vi "TableGluing.vi"() -> ()   [LabVIEW 2015]
uses:
  GlobalPath.vi
  GlobalData.vi
  GlobalVi.vi
panel:
  in  "Done with gluing?":bool
  in  "ptfe 7":bool caption="Remove the parchment covers from on top of the PCBs"
  in  "ptfe 6":bool caption="Remove the frames, cooling bars and honeycombs from on top of \nthe PCBs on the table"
  in  "Done?":bool
  in  "ptfe 5":bool caption="Open the vi with the gluing instructions"
  in  "ptfe 4":bool caption="Position the cartridge on the glue machine housing"
  in  "ptfe 3":bool caption="Mount the dispenser on the glue cartridge"
  in  "ptfe 2":bool caption="Position parchment covers to protect the reference plates and external \nparts of the 5 PCBs"
  # "Gluing on Table"
  # "Start gluing process"
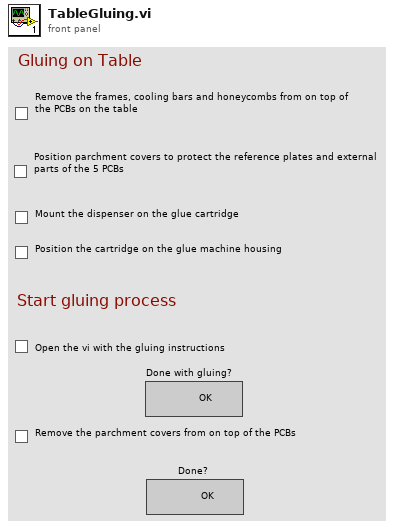
[diagram p1: front panel]
types:
  T1 = enum16{"open", "replace", "create", "open or create", "replace or create", "replace or create with confirmation"}
  T2 = enum32{"Bad", "Idle", "Run top level", "Running"}
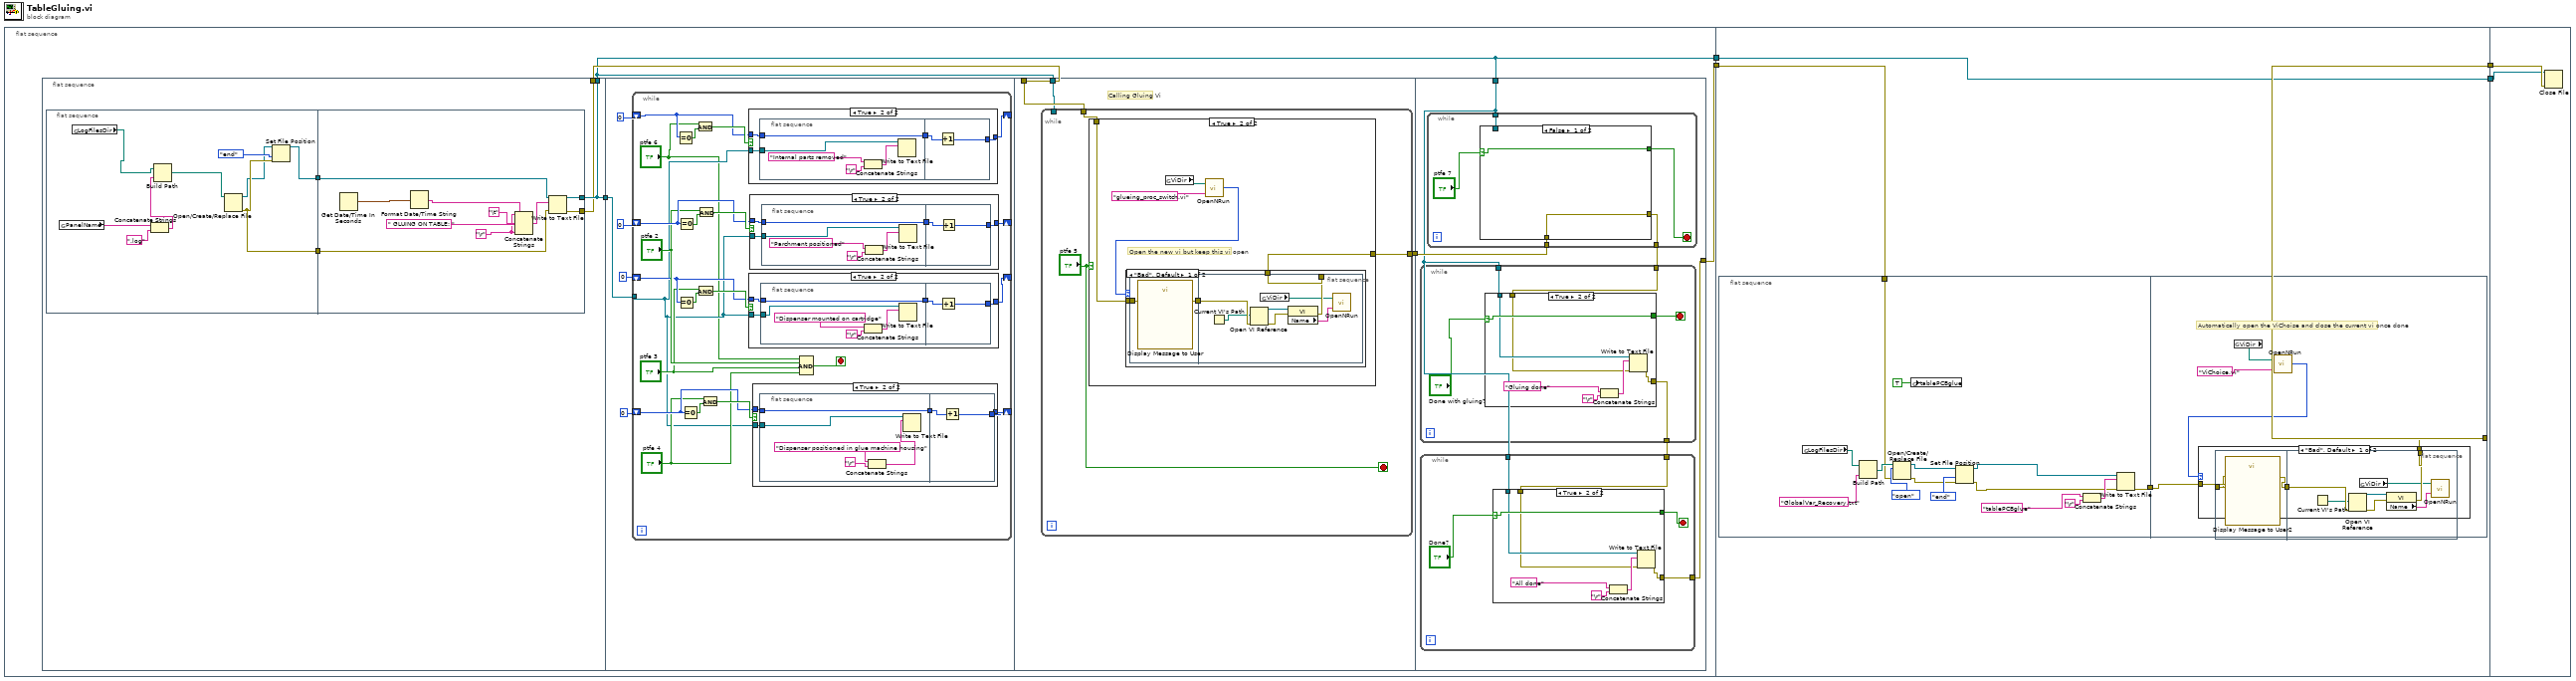
[diagram p0: block diagram]
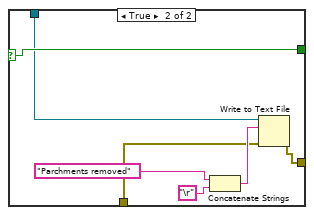
[diagram p9: hidden frame]
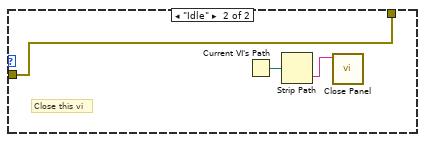
[diagram p11: hidden frame]
diagram:
  n1 = flat-sequence {
    tunnel: [w6] -> w3
    tunnel: [w5] -> w1
    tunnel: [w183] -> w4
    tunnel: w3 -> [w182]
    tunnel: [w182] -> w2
    tunnel: w1 -> [w180]
    tunnel: w4 -> [w220]
    tunnel: w2 -> [w219]
    frame #0 {
      n2 = flat-sequence {
        tunnel: [w12] -> w9
        tunnel: [w12] -> w6
        tunnel: [w11] -> w8
        tunnel: w9 -> [w37]
        tunnel: w8 -> [w110]
        tunnel: w6 -> [w108]
        tunnel: [w109] -> w7
        tunnel: [w134] -> w5
        tunnel: w7 -> [w137]
        tunnel: w6 -> [w133]
        frame #0 {
          n3 = flat-sequence {
            tunnel: [w15] -> w13
            tunnel: [w17] -> w10
            tunnel: w13 -> [w28]
            tunnel: [w27] -> w12
            tunnel: [w26] -> w11
            tunnel: w10 -> [w25]
            frame #0 {
              n4 = global read "GlobalData.vi" "PanelName"() -> (w21:string)
              n5 = global read "GlobalPath.vi" "LogFilesDir"() -> (w14:path)
              n6 = Concatenate Strings(w21, ".log") -> (w20:string)
              n7 = Build Path(base path=w14, name or relative path=w20) -> (appended path=w19:path)
              n8 = Open/Create/Replace File(file path (use dialog)=w19) -> (refnum out=w16:refnum<file>, error out=w17:errorcluster)  [unwired: 5 in, 1 out]
              n9 = Set File Position(refnum=w16, from (0:start)=enum16{"start", "end", "current"}."end", error in=w17) -> (refnum out=w15:refnum<file>)  [unwired: 1 in, 1 out]
            }
            frame #1 {
              w23 = "\r"
              n10 = Get Date/Time In Seconds() -> (seconds since 1Jan1904=w24:timestamp)
              n11 = Format Date/Time String(seconds (now)=w24) -> (date/time string=w30:string)  [unwired: 2 in]
              n12 = Concatenate Strings(w23, w30, "\t", " GLUING ON TABLE: ", w23) -> (w29:string)
              n13 = Write to Text File(file (use dialog)=w28, text=w29, error in=w25) -> (refnum out=w27:refnum<file>, error out=w26:errorcluster)  [unwired: 1 in, 1 out]
            }
          }
        }
        frame #1 {
          n14 = while {
            tunnel: w37 -> [w39]
            shift-right: [w55] -> _
            shift-left: 0 -> [w56]
            shift-right: [w46] -> _
            shift-left: 0 -> [w51]
            shift-right: [w45] -> _
            shift-left: 0 -> [w47]
            shift-right: [w41] -> _
            shift-left: 0 -> [w40]
            stop <- w59 stop-if-true
            n15 = Equal To 0?(x=w40) -> (x = 0?=w43:bool)
            n16 = Equal To 0?(x=w51) -> (x = 0?=w53:bool)
            n17 = Equal To 0?(x=w56) -> (x = 0?=w58:bool)
            n18 = Equal To 0?(x=w47) -> (x = 0?=w49:bool)
            n19 = And(x="ptfe 6", y=w43) -> (x .and. y?=w42:bool)
            n20 = And(x="ptfe 3", y=w53) -> (x .and. y?=w52:bool)
            n21 = And(x="ptfe 2", y=w58) -> (x .and. y?=w57:bool)
            n22 = And(x="ptfe 4", y=w49) -> (x .and. y?=w48:bool)
            n23 = case shown="True" w42 {
              tunnel: w39 -> [_ w64]
              tunnel: w40 -> [w60 w62]
              tunnel: [w60 w61] -> w41
              frame False {
              }
              frame True {
                n24 = flat-sequence {
                  tunnel: w64 -> [w66]
                  tunnel: [w65] -> w63
                  tunnel: w62 -> [w65]
                  tunnel: w63 -> [w71]
                  tunnel: [w70] -> w61
                  frame #0 {
                    n25 = Concatenate Strings("Internal parts removed", "\r") -> (w69:string)
                    n26 = Write to Text File(file (use dialog)=w66, text=w69) -> ()  [unwired: 2 in, 3 out]
                  }
                  frame #1 {
                    n27 = Increment(x=w71) -> (x+1=w70:i32)
                  }
                }
              }
            }
            n28 = case shown="True" w52 {
              tunnel: w39 -> [_ w88]
              tunnel: w51 -> [w84 w86]
              tunnel: [w84 w85] -> w46
              frame False {
              }
              frame True {
                n29 = flat-sequence {
                  tunnel: w88 -> [w91]
                  tunnel: [w90] -> w87
                  tunnel: w86 -> [w90]
                  tunnel: w87 -> [w95]
                  tunnel: [w94] -> w85
                  frame #0 {
                    n30 = Concatenate Strings("Dispenser mounted on cartridge", "\r") -> (w93:string)
                    n31 = Write to Text File(file (use dialog)=w91, text=w93) -> ()  [unwired: 2 in, 3 out]
                  }
                  frame #1 {
                    n32 = Increment(x=w95) -> (x+1=w94:i32)
                  }
                }
              }
            }
            n33 = case shown="True" w57 {
              tunnel: w39 -> [_ w100]
              tunnel: w56 -> [w96 w98]
              tunnel: [w96 w97] -> w55
              frame False {
              }
              frame True {
                n34 = flat-sequence {
                  tunnel: w100 -> [w102]
                  tunnel: [w101] -> w99
                  tunnel: w98 -> [w101]
                  tunnel: w99 -> [w107]
                  tunnel: [w106] -> w97
                  frame #0 {
                    n35 = Concatenate Strings("Parchment positioned", "\r") -> (w105:string)
                    n36 = Write to Text File(file (use dialog)=w102, text=w105) -> ()  [unwired: 2 in, 3 out]
                  }
                  frame #1 {
                    n37 = Increment(x=w107) -> (x+1=w106:i32)
                  }
                }
              }
            }
            n38 = case shown="True" w48 {
              tunnel: w39 -> [_ w76]
              tunnel: w47 -> [w72 w74]
              tunnel: [w72 w73] -> w45
              frame False {
              }
              frame True {
                n39 = flat-sequence {
                  tunnel: w76 -> [w79]
                  tunnel: [w78] -> w75
                  tunnel: w74 -> [w78]
                  tunnel: w75 -> [w83]
                  tunnel: [w82] -> w73
                  frame #0 {
                    n40 = Concatenate Strings("Dispenser positioned in glue machine housing", "\r") -> (w81:string)
                    n41 = Write to Text File(file (use dialog)=w79, text=w81) -> ()  [unwired: 2 in, 3 out]
                  }
                  frame #1 {
                    n42 = Increment(x=w83) -> (x+1=w82:i32)
                  }
                }
              }
            }
            n43 = Compound Arithmetic op=AND("ptfe 6", "ptfe 2", "ptfe 3", "ptfe 4") -> (w59:bool)
          }
        }
        frame #2 {
          # "Calling Gluing Vi"
          n44 = while {
            tunnel: w110 -> [w113]
            tunnel: [w112] -> w109
            tunnel: w108 -> [_]
            stop <- "ptfe 5" stop-if-true
            n45 = case shown="True" "ptfe 5" {
              tunnel: w113 -> [w114 w116]
              tunnel: [w114 w115] -> w112
              frame False {
              }
              frame True {
                # "Open the new vi but keep this vi open"
                n46 = global read "GlobalPath.vi" "ViDir"() -> (w119:path)
                n47 = call "OpenNRun.vi"("VI name"="glueing_proc_switch.vi", "ViDirPath"=w119) -> ("Execution:State"=w118:T2)
                n48 = case shown="\"Bad\", Default" w118 {
                  tunnel: [w122 w132] -> w115
                  tunnel: w116 -> [w121 w132]
                  frame "Bad", Default {
                    n49 = flat-sequence {
                      tunnel: w121 -> [w123]
                      tunnel: [w124] -> w120
                      tunnel: [w128] -> w122
                      tunnel: w120 -> [w127]
                      frame #0 {
                        n50 = call "Display Message to User"("error in (no error)"=w123) -> ("error out"=w124:errorcluster)  [unwired: 9 in, 1 out]
                      }
                      frame #1 {
                        n51 = Current VI's Path() -> (path=w125:path)
                        n52 = Open VI Reference(vi path=w125, error in (no error)=w127) -> (vi reference=w131:refnum<vi>, error out=w130:errorcluster)  [unwired: 4 in]
                        n53 = global read "GlobalPath.vi" "ViDir"() -> (w126:path)
                        n54 = property class="VI"(reference=w131, error in=w130) -> (error out=w128:errorcluster, "Name"=w129:string)  [unwired: 1 out]
                        n55 = call "OpenNRun.vi"("VI name"=w129, "ViDirPath"=w126) -> ()  [unwired: 1 out]
                      }
                    }
                  }
                  frame "Idle" {
                    # "Program opened"
                  }
                }
              }
            }
          }
        }
        frame #3 {
          n56 = while {
            tunnel: w133 -> [w156]
            tunnel: w137 -> [w155]
            tunnel: [w154] -> w136
            stop <- w152 stop-if-true
            n57 = case shown="False" "ptfe 7" {
              selector: "ptfe 7" -> [w158 w162]
              tunnel: [w158 w162] -> w152
              tunnel: w156 -> [_ w161]
              tunnel: [w157 w160] -> w154
              tunnel: w155 -> [w157 w159]
              frame False {
              }
              frame True {
                n58 = Concatenate Strings("Parchments removed", "\r") -> (w165:string)
                n59 = Write to Text File(file (use dialog)=w161, text=w165, error in=w159) -> (error out=w160:errorcluster)  [unwired: 1 in, 2 out]
              }
            }
          }
          n60 = while {
            tunnel: w133 -> [w169]
            tunnel: w136 -> [w168]
            tunnel: [w167] -> w135
            stop <- w170 stop-if-true
            n61 = case shown="True" "Done with gluing?" {
              selector: "Done with gluing?" -> [w172 w176]
              tunnel: [w172 w176] -> w170
              tunnel: w169 -> [_ w175]
              tunnel: w168 -> [w171 w174]
              tunnel: [w171 w173] -> w167
              frame False {
              }
              frame True {
                n62 = Concatenate Strings("Gluing done", "\r") -> (w179:string)
                n63 = Write to Text File(file (use dialog)=w175, text=w179, error in=w174) -> (error out=w173:errorcluster)  [unwired: 1 in, 2 out]
              }
            }
          }
          n64 = while {
            tunnel: w135 -> [w141]
            tunnel: [w140] -> w134
            tunnel: w133 -> [w139]
            stop <- w142 stop-if-true
            n65 = case shown="True" "Done?" {
              selector: "Done?" -> [w144 w148]
              tunnel: [w144 w148] -> w142
              tunnel: w139 -> [_ w147]
              tunnel: w141 -> [w143 w146]
              tunnel: [w143 w145] -> w140
              frame False {
              }
              frame True {
                n66 = Concatenate Strings("All done", "\r") -> (w151:string)
                n67 = Write to Text File(file (use dialog)=w147, text=w151, error in=w146) -> (error out=w145:errorcluster)  [unwired: 1 in, 2 out]
              }
            }
          }
        }
      }
    }
    frame #1 {
      n68 = flat-sequence {
        tunnel: [w187] -> w181
        tunnel: w180 -> [w186]
        tunnel: [w200] -> w183
        tunnel: w181 -> [w199]
        frame #0 {
          n69 = global read "GlobalPath.vi" "LogFilesDir"() -> (w184:path)
          n70 = Build Path(base path=w184, name or relative path="GlobalVar_Recovery.txt") -> (appended path=w196:path)
          n71 = Open/Create/Replace File(file path (use dialog)=w196, error in=w186, operation (0:open)=T1."open") -> (refnum out=w192:refnum<file>, error out=w193:errorcluster)  [unwired: 3 in, 1 out]
          n72 = global write "GlobalVi.vi" "tablePCBglue"(TRUE) -> ()
          n73 = Set File Position(refnum=w192, from (0:start)=enum16{"start", "end", "current"}."end", error in=w193) -> (refnum out=w189:refnum<file>, error out=w188:errorcluster)  [unwired: 1 in]
          n74 = Concatenate Strings("tablePCBglue", "\r") -> (w191:string)
          n75 = Write to Text File(file (use dialog)=w189, text=w191, error in=w188) -> (error out=w187:errorcluster)  [unwired: 1 in, 2 out]
        }
        frame #1 {
          # "Automatically open the ViChoise and close the current vi once done"
          n76 = global read "GlobalPath.vi" "ViDir"() -> (w203:path)
          n77 = call "OpenNRun.vi"("VI name"="ViChoice.vi", "ViDirPath"=w203) -> ("Execution:State"=w202:T2)
          n78 = case shown="\"Bad\", Default" w202 {
            tunnel: [w206 w218] -> w200
            tunnel: w199 -> [w205 w218]
            frame "Bad", Default {
              n79 = flat-sequence {
                tunnel: w205 -> [w208]
                tunnel: [w207] -> w204
                tunnel: [w212] -> w206
                tunnel: w204 -> [w211]
                frame #0 {
                  n80 = call "Display Message to User2"("error in (no error)"=w208) -> ("error out"=w207:errorcluster)  [unwired: 9 in, 1 out]
                }
                frame #1 {
                  n81 = Current VI's Path() -> (path=w209:path)
                  n82 = Open VI Reference(vi path=w209, error in (no error)=w211) -> (vi reference=w215:refnum<vi>, error out=w214:errorcluster)  [unwired: 4 in]
                  n83 = global read "GlobalPath.vi" "ViDir"() -> (w210:path)
                  n84 = property class="VI"(reference=w215, error in=w214) -> (error out=w212:errorcluster, "Name"=w213:string)  [unwired: 1 out]
                  n85 = call "OpenNRun.vi"("VI name"=w213, "ViDirPath"=w210) -> ()  [unwired: 1 out]
                }
              }
            }
            frame "Idle" {
              # "Close this vi"
              n86 = Current VI's Path() -> (path=w217:path)
              n87 = Strip Path(path=w217) -> (name=w216:string)  [unwired: 1 out]
              n88 = call <vilib>:"Close Panel.vi"("VI name"=w216) -> ()  [unwired: 10 in, 1 out]
            }
          }
        }
      }
    }
    frame #2 {
      n89 = Close File(refnum=w219, error in=w220) -> ()  [unwired: 2 out]
    }
  }
